vi "test6-RegisterStatusFromNonCSM.vi"(8 "error in (no error)":errorcluster, 11 "TestCase in":refnum<class "testcase-CSMBroadcast.lvclass">) -> (0 "error out":errorcluster, 3 "TestCase out":refnum<class "testcase-CSMBroadcast.lvclass">)   [LabVIEW 2017, in "testcase-CSMBroadcast.lvclass"]
uses:
  testcase-CSMBroadcast.lvclass
  <vilib>/addons/_JKI Toolkits/VI Tester/TestCase.llb/TestCase.lvclass
  src/user.lib/_NEVSTOP/Communicable State Machine(CSM)/Communicable State Machine.lvlib
  C:/Program Files (x86)/National Instruments/LabVIEW 2017/vi.lib/addons/_JKI Toolkits/VI Tester/TestCase.llb/TestCase.lvclass
panel:
  out "error out 3":errorcluster
  out "error out 2":errorcluster
  out "LoopCount":i32
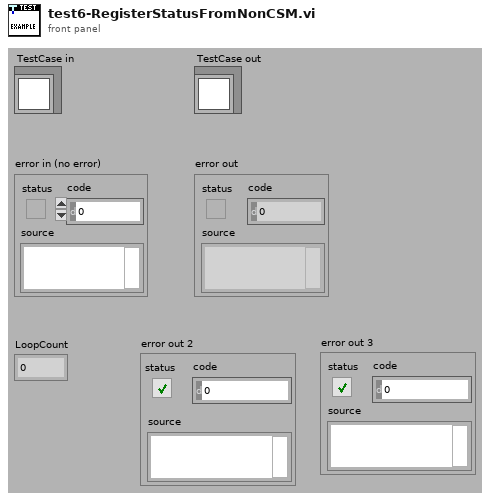
[diagram p1: front panel]
types:
  T1 = cluster{"ModuleName":string, "Status":string, "Arguments":string}
  T2 = cluster{"cluster":cluster{"ModuleName":string, "Status":string, "Arguments":string}}
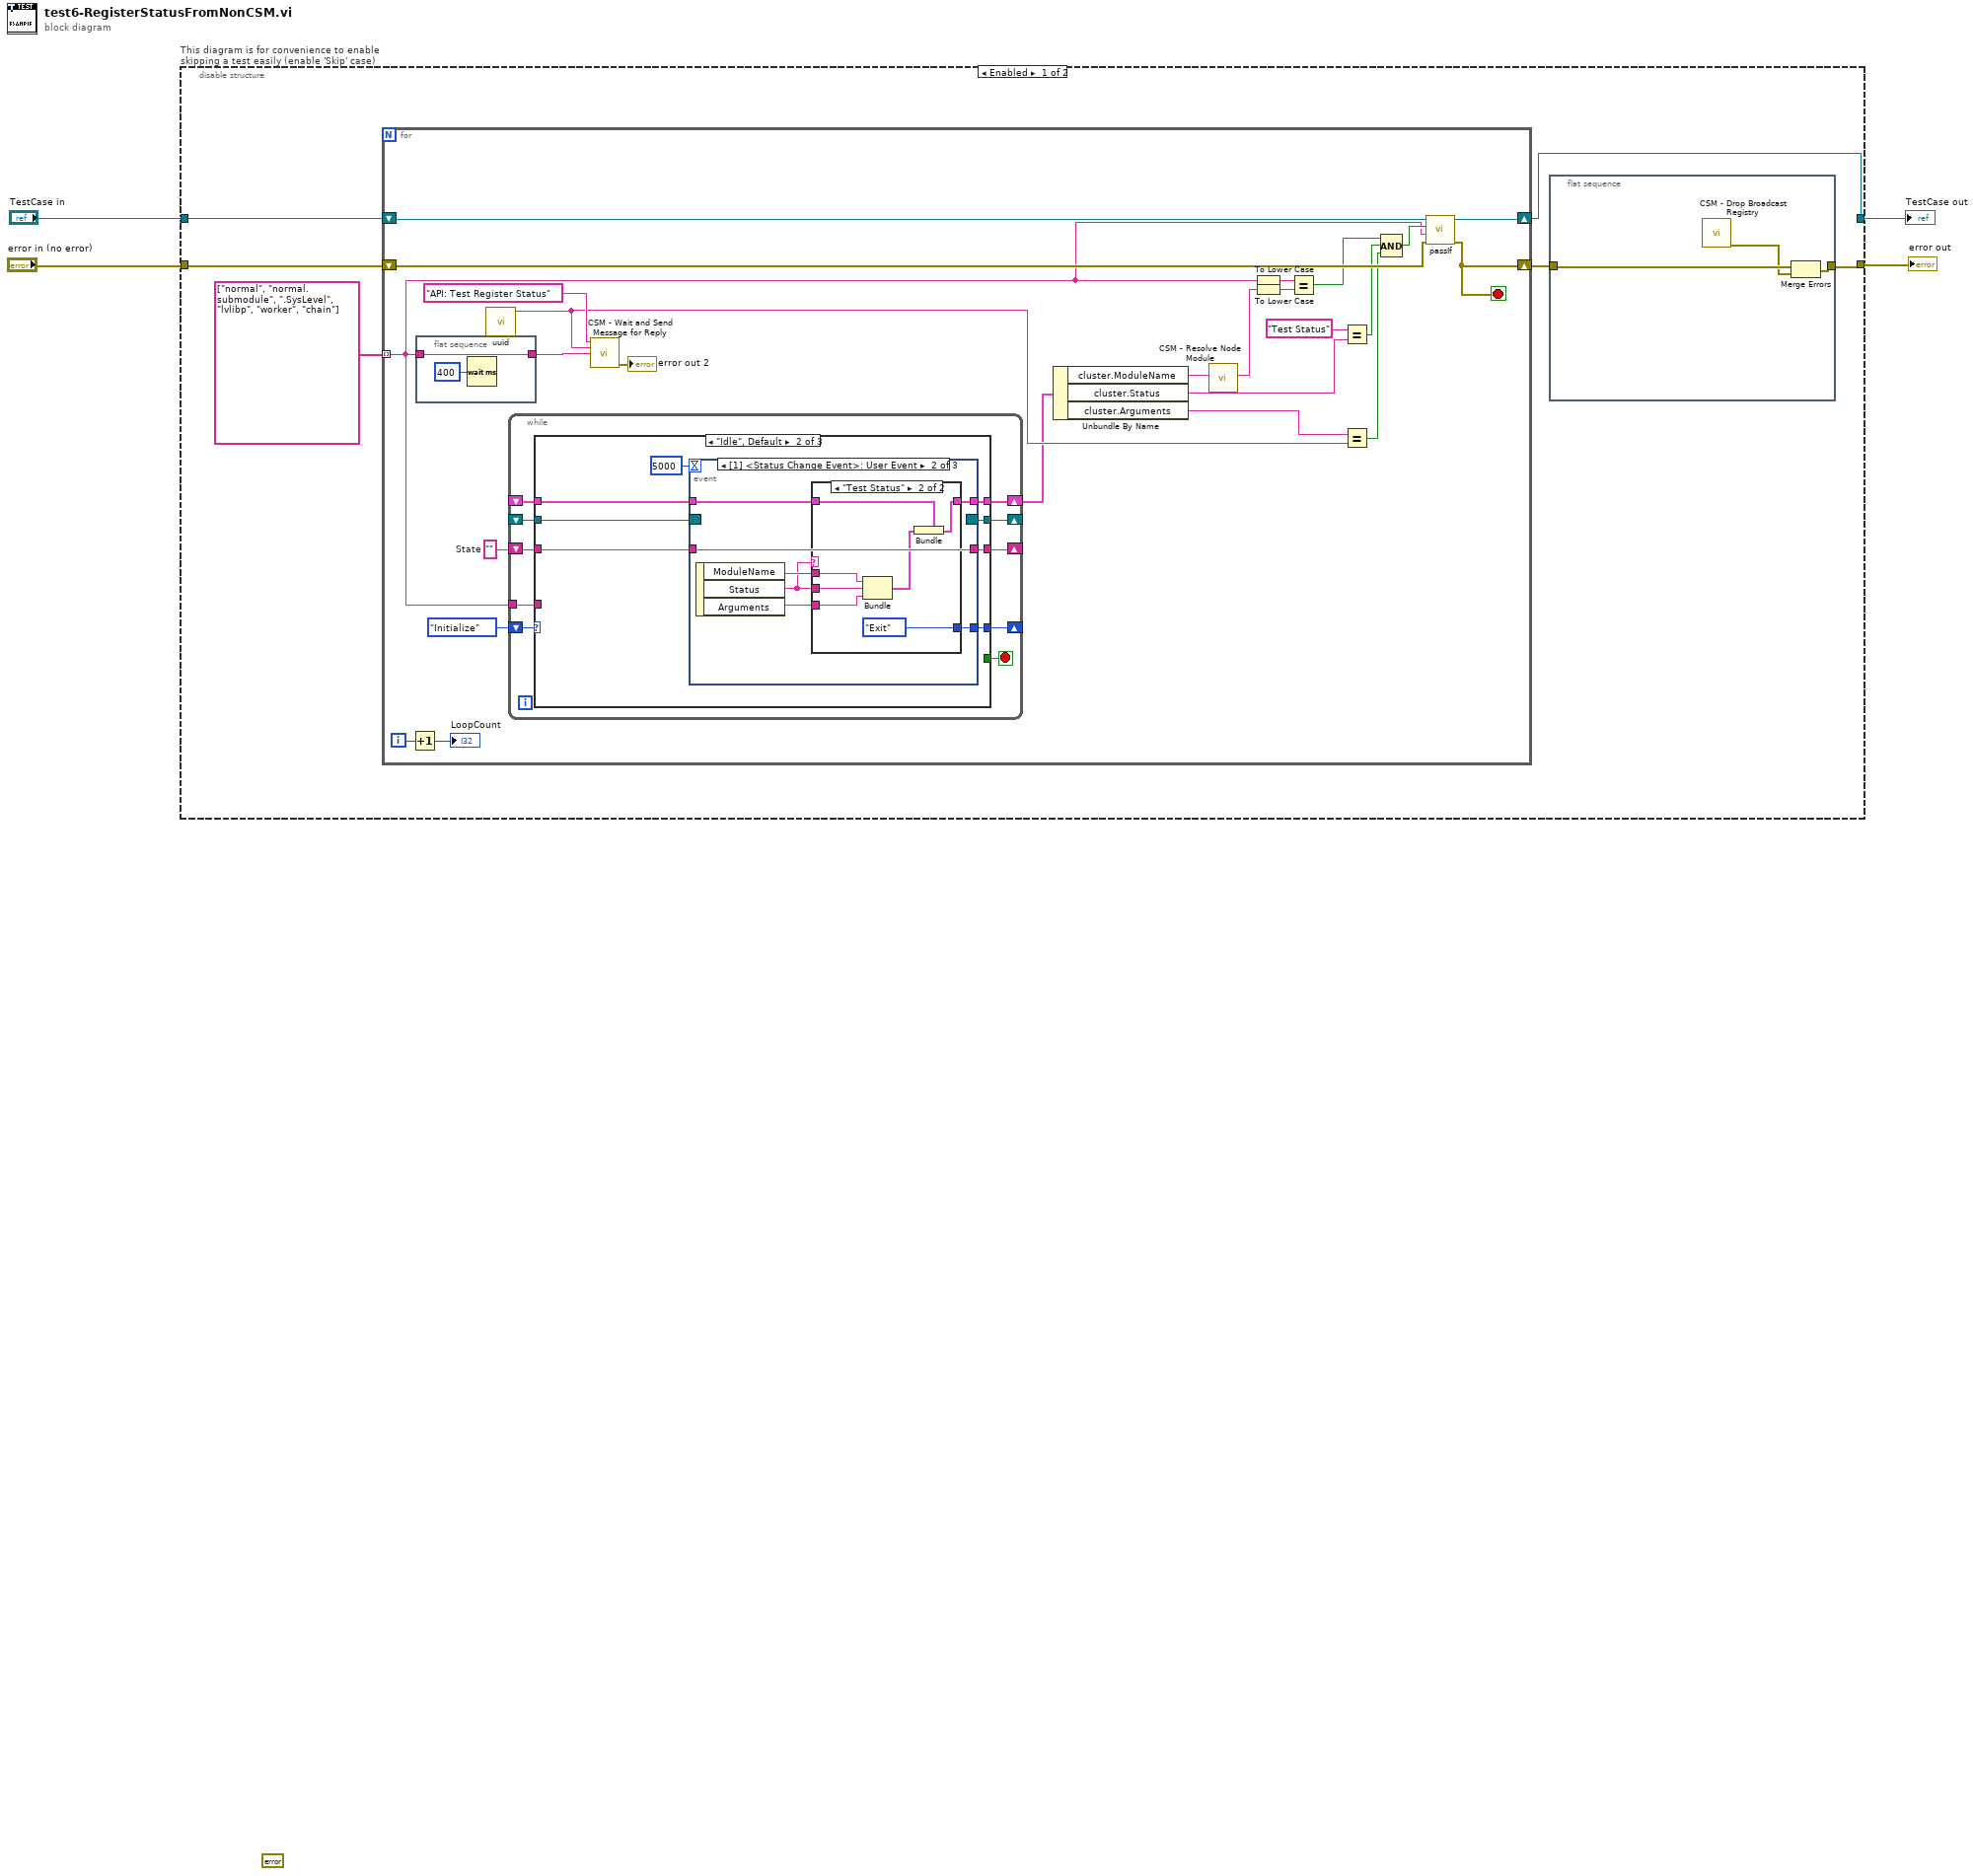
[diagram p0: block diagram]
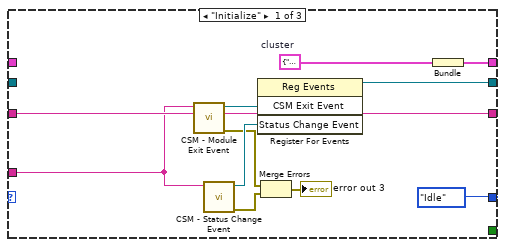
[diagram p2: hidden frame]
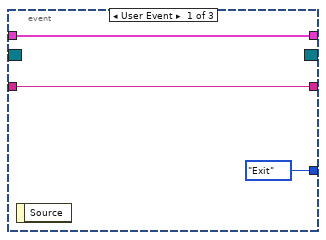
[diagram p3: hidden frame]
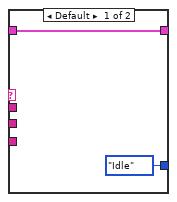
[diagram p4: hidden frame]
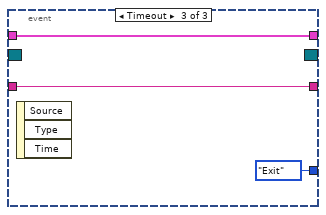
[diagram p5: hidden frame]
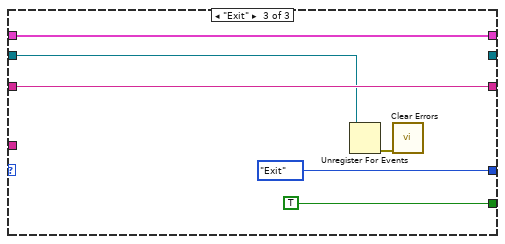
[diagram p6: hidden frame]
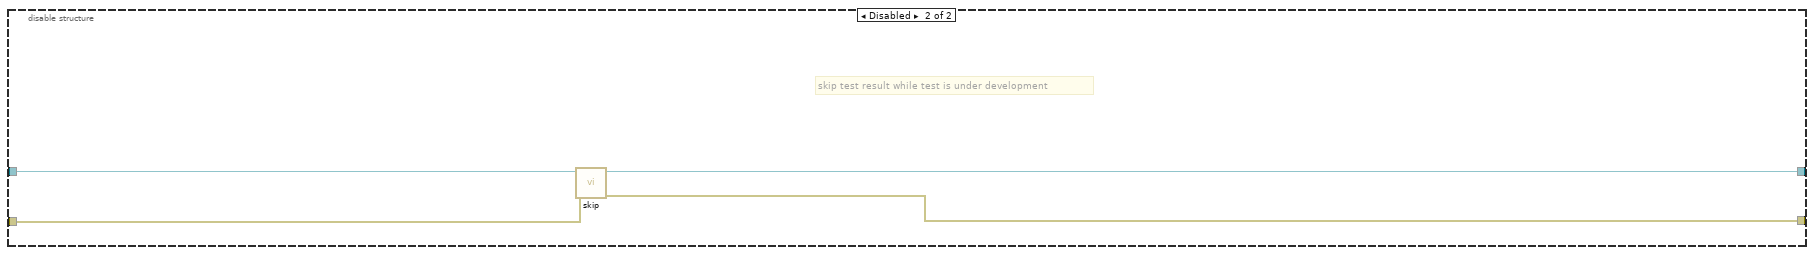
[diagram p7: hidden frame]
diagram:
  (unwired) errorcluster {"status"=FALSE, "code"=0, "source"=""} ("error out")
  n1 = disable-structure "This diagram is for convenience to enable skipping a test easily (enable 'Skip' case)" shown="Enabled" {
    disable-tunnel: "TestCase in" -> [w10 w101]
    disable-tunnel: [w6 w99] -> w2
    disable-tunnel: [w5 w100] -> w1
    disable-tunnel: "error in (no error)" -> [w9 w98]
    frame Enabled {
      n2 = for {
        shift-right: [w29] -> w6
        shift-left: w10 -> [w30]
        tunnel: string[] ["normal", "normal.submodule", ".SysLevel", "lvlibp", "worker", "chain"] -> [w15] mode=indexing
        shift-right: [w20] -> w7
        shift-left: w9 -> [w28]
        i -> [w23]
        stop <- w20 stop-if-true
        w37 = ""  # State
        n3 = Increment(x=w23) -> (x+1=→"LoopCount":i32)
        n4 = flat-sequence {
          tunnel: w15 -> [w40]
          tunnel: [w40] -> w35
          frame #0 {
            n5 = Wait (ms)(milliseconds to wait=u32 400) -> ()  [unwired: 1 out]
          }
        }
        n6 = call "uuid.vi"() -> ("UUID"=w32:string)  [unwired: 11 in]
        n7 = while {
          shift-right: [w49] -> _
          shift-left: enum16{"Idle", "Initialize", "Exit"}."Initialize" -> [w50]
          shift-right: [w46] -> _
          shift-left: w37 -> [w47]
          shift-right: [w45] -> _
          shift-left: _ -> [w44]
          shift-right: [w43] -> w19
          shift-left: _ -> [w42]
          tunnel: w15 -> [w41]
          stop <- w48 stop-if-true
          n8 = case shown="\"Idle\", Default" w50 {
            tunnel: [enum16{"Idle", "Initialize", "Exit"}."Idle" w69 enum16{"Idle", "Initialize", "Exit"}."Exit"] -> w49
            tunnel: [_ _ TRUE] -> w48
            tunnel: w47 -> [w60 w67 w95]
            tunnel: [w60 w68 w95] -> w46
            tunnel: [w58 w65 _] -> w45
            tunnel: w44 -> [_ w66 w94]
            tunnel: [w57 w63 w92] -> w43
            tunnel: w42 -> [_ w64 w92]
            tunnel: w41 -> [w55 _ _]
            frame "Initialize" {
              w54 = T1 {"ModuleName"="", "Status"="", "Arguments"=""}  # cluster
              n9 = call "CSM - Module Exit Event.vi"("Name (\"\" to Use UUID) In"=w55) -> ("error out"=w53:errorcluster, "CSM Exit Event"=w59:refnum<user-event>)  [unwired: 8 in, 1 out]
              n10 = call "CSM - Status Change Event.vi"("CSM Module"=w55) -> ("error out"=w52:errorcluster, "Status Change Event"=w56:refnum<user-event>)  [unwired: 8 in, 1 out]
              n11 = register-events(w59, w56) -> (reference out=w58:refnum<event-registration>)  [unwired: 2 in, 1 out]
              n12 = Merge Errors(w53, w52) -> (→"error out 3":errorcluster)
              n13 = Bundle("cluster"=w54) -> (w57:T2)  [unwired: 1 in]
            }
            frame "Idle", Default {
              n14 = event shown="[1] <Status Change Event>: User Event" {
                selector: w66 -> [_ _ _]
                dyn-events: [_ _ _] -> w65
                timeout: 5000 -> [_ _ _]
                tunnel: [enum16{"Idle", "Initialize", "Exit"}."Exit" w78 enum16{"Idle", "Initialize", "Exit"}."Exit"] -> w69
                tunnel: w67 -> [w72 w79 w91]
                tunnel: [w72 w79 w91] -> w68
                tunnel: w64 -> [w70 w75 w90]
                tunnel: [w70 w74 w90] -> w63
                event User Event {
                  n15 = event-data() -> ()  [unwired: 1 in, 1 out]
                }
                event User Event {
                  n16 = event-data() -> ("ModuleName"=w77:string, "Status"=w73:string, "Arguments"=w76:string)  [unwired: 1 in]
                  n17 = case shown="\"Test Status\"" w73 {
                    tunnel: [enum16{"Idle", "Initialize", "Exit"}."Idle" enum16{"Idle", "Initialize", "Exit"}."Exit"] -> w78
                    tunnel: w77 -> [_ w87]
                    tunnel: w73 -> [_ w86]
                    tunnel: w76 -> [_ w85]
                    tunnel: w75 -> [w81 w84]
                    tunnel: [w81 w82] -> w74
                    frame Default {
                    }
                    frame "Test Status" {
                      n18 = Bundle("ModuleName"=w87, "Status"=w86, "Arguments"=w85) -> (w83:T1)  [unwired: 1 in]
                      n19 = Bundle(cluster=w84, "cluster"=w83) -> (w82:T2)
                    }
                  }
                }
                event Timeout {
                  n20 = event-data() -> ()  [unwired: 1 in, 3 out]
                }
              }
            }
            frame "Exit" {
              n21 = Unregister For Events(event registration refnum=w94) -> (error out=w93:errorcluster)  [unwired: 1 in]
              n22 = call <vilib>:"Clear Errors.vi"("error in (no error)"=w93) -> ()  [unwired: 5 in, 2 out]
            }
          }
        }
        n23 = call "CSM - Wait and Send Message for Reply.vi"("State"="API: Test Register Status", "Arguments (\"\")"=w32, "Target Module"=w35) -> ("error out"=→"error out 2":errorcluster)  [unwired: 10 in, 2 out]
        n24 = Unbundle By Name(w19) -> ("cluster.ModuleName"=w17:string, "cluster.Status"=w33:string, "cluster.Arguments"=w31:string)
        n25 = call "CSM - Resolve Node Module.vi"("Node Name"=w17) -> ("CSM Module Name"=w14:string)  [unwired: 10 in]
        n26 = To Lower Case(string=w15) -> (all lower case string=w18:string)
        n27 = To Lower Case(string=w14) -> (all lower case string=w16:string)
        n28 = Equal?(x=w18, y=w16) -> (x = y?=w27:bool)
        n29 = Equal?(x="Test Status" ("State"), y=w33) -> (x = y?=w26:bool)
        n30 = Equal?(x=w31, y=w32) -> (x = y?=w25:bool)
        n31 = Compound Arithmetic op=AND(w27, w26, w25) -> (w24:bool)
        n32 = call-dynamic "passIf.vi"("error in (no error)"=w28, "message (\"\")"=w15, "pass"=w24, "TestCase in"=w30) -> ("error out"=w20:errorcluster, "TestCase out"=w29:refnum<class "testcase-CSMBroadcast.lvclass">)  [unwired: 6 in]
      }
      n33 = flat-sequence {
        tunnel: w7 -> [w13]
        tunnel: [w12] -> w5
        frame #0 {
          n34 = call "CSM - Drop Broadcast Registry.vi"() -> ("error out"=w11:errorcluster)  [unwired: 15 in]
          n35 = Merge Errors(w13, w11) -> (w12:errorcluster)
        }
      }
    }
    frame Disabled {
      # "skip test result while test is under development"
      n36 = call <vilib>:"skip.vi"("error in (no error)"=w98, "TestCase in"=w101) -> ("error out"=w100:errorcluster, "TestCase out"=w99:refnum<class "testcase-CSMBroadcast.lvclass">)  [unwired: 8 in]
    }
  }
  "error out" <- w1
  "TestCase out" <- w2
